vi "Generate PXIe-7820R Bitfile Path.vi"() -> (0 "Bitfile Path":path)   [LabVIEW 2018, in "FPGA Addon Load And Parse Bitfile Unit Tests.lvclass"]
uses:
  FPGA Addon Load And Parse Bitfile Unit Tests.lvclass
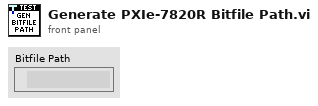
[diagram p1: front panel]
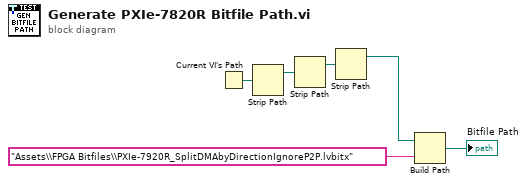
[diagram p0: block diagram]
diagram:
  n1 = Current VI's Path() -> (path=w6:path)
  n2 = Strip Path(path=w6) -> (stripped path=w5:path)  [unwired: 1 out]
  n3 = Strip Path(path=w5) -> (stripped path=w4:path)  [unwired: 1 out]
  n4 = Strip Path(path=w4) -> (stripped path=w3:path)  [unwired: 1 out]
  n5 = Build Path(base path=w3, name or relative path="Assets\\FPGA Bitfiles\\PXIe-7920R_SplitDMAbyDirectionIgnoreP2P.lvbitx") -> (appended path=→"Bitfile Path":path)
